vi "Make K-Points File.vi"() -> ()   [LabVIEW 2010]
uses:
  <vilib>/Analysis/NI_AALPro.lvlib
  <vilib>/Analysis/_algsub.llb/Real Vector Norm.vi
panel:
  out "K-Points File":string
  in  "Tab Control":enum32{"Automatic", "Manual"}(tab)
  in  "|G| Factor":dbl
  in  "Auto Type":T1(radio)
  in  "Shift":dbl[](array[numeric])
  in  "Lattice vector a":dbl[](array[numeric])
  in  "Lattice vector b":dbl[](array[numeric])
  in  "Lattice vector c":dbl[](array[numeric])
  in  "Symmetry":enum32{"High-Symmetry", "L-G-X", "Manual Mesh"}(radio)
  in  "# Points between":i32
  in  "Manual Type":enum32{"Reciprocal", "Cartesian"}(radio)
  in  "K-point Mesh":T2(array[cluster])
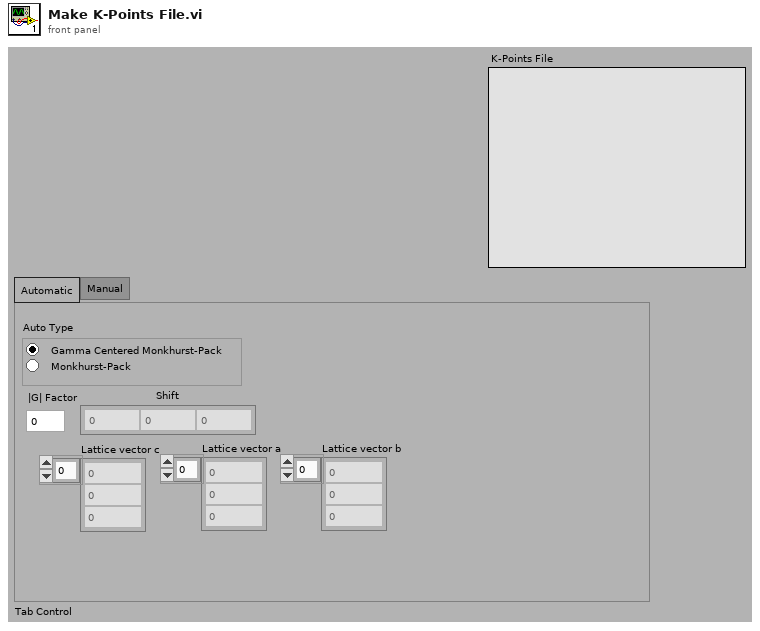
[diagram p1: front panel]
types:
  T1 = enum32{"Gamma Centered Monkhurst-Pack", "Monkhurst-Pack"}
  T2 = cluster{"Start":dbl, "End":dbl, "Step or #pts":dbl, "Style":enum16{"Linear Step", "Linear Pts", "Log Pts"}, "Parameter":string}[]
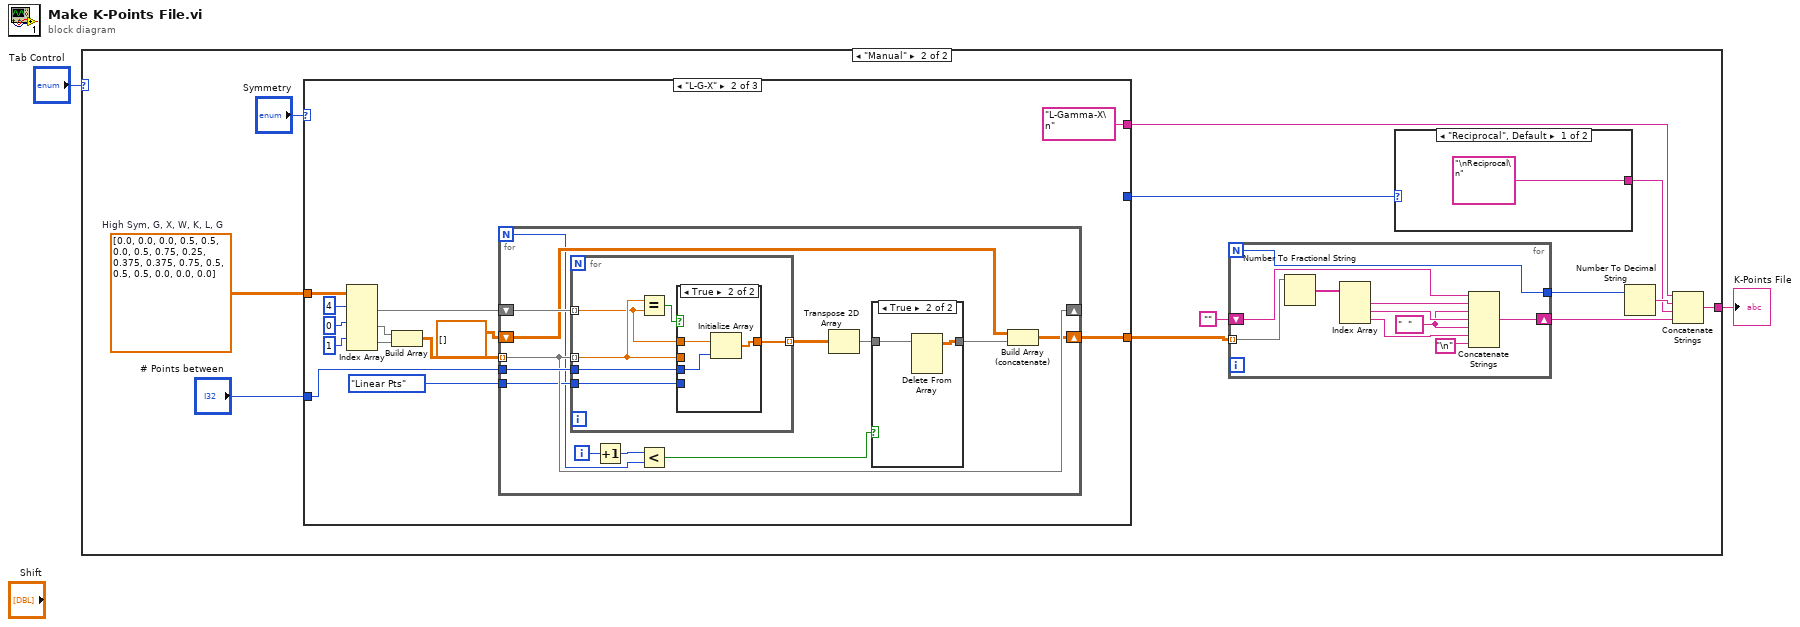
[diagram p0: block diagram]
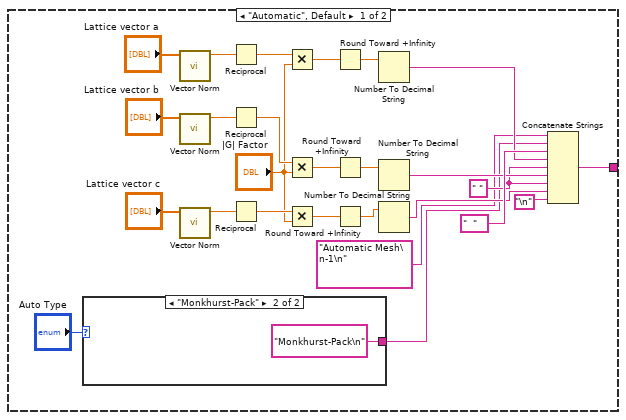
[diagram p2: hidden frame]
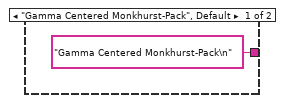
[diagram p3: hidden frame]
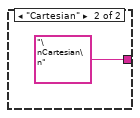
[diagram p4: hidden frame]
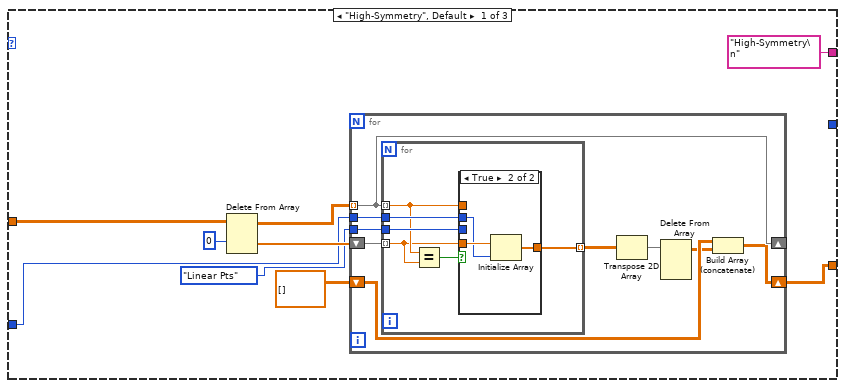
[diagram p5: hidden frame]
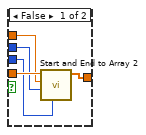
[diagram p6: hidden frame]
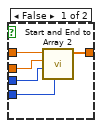
[diagram p8: hidden frame]
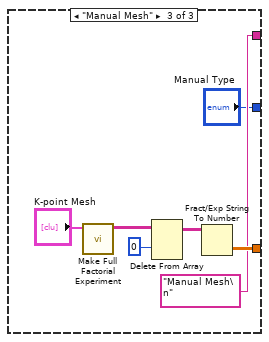
[diagram p9: hidden frame]
diagram:
  n1 = case shown="\"Manual\"" "Tab Control" {
    tunnel: [w7 w31] -> w1
    frame "Automatic", Default {
      w12 = " " ("string")
      n2 = case shown="\"Monkhurst-Pack\"" "Auto Type" {
        tunnel: ["Gamma Centered Monkhurst-Pack\n" "Monkhurst-Pack\n"] -> w8
        frame "Gamma Centered Monkhurst-Pack", Default {
        }
        frame "Monkhurst-Pack" {
        }
      }
      n3 = call-poly <vilib>:"Vector Norm.vi"("Input Vector"="Lattice vector a") -> ("norm"=w26:dbl)  [unwired: 9 in, 1 out]
      n4 = call-poly <vilib>:"Vector Norm.vi"("Input Vector"="Lattice vector b") -> ("norm"=w23:dbl)  [unwired: 9 in, 1 out]
      n5 = call-poly <vilib>:"Vector Norm.vi"("Input Vector"="Lattice vector c") -> ("norm"=w20:dbl)  [unwired: 9 in, 1 out]
      n6 = Reciprocal(x=w26) -> (1/x=w27:dbl)
      n7 = Reciprocal(x=w23) -> (1/x=w22:dbl)
      n8 = Reciprocal(x=w20) -> (1/x=w21:dbl)
      n9 = Multiply(x=w27, y="|G| Factor") -> (x*y=w25:dbl)
      n10 = Multiply(x=w22, y="|G| Factor") -> (x*y=w24:dbl)
      n11 = Multiply(x=w21, y="|G| Factor") -> (x*y=w19:dbl)
      n12 = Round Toward +Infinity(x=w25) -> (ceil(x): smallest int >= x=w18:dbl)
      n13 = Round Toward +Infinity(x=w24) -> (ceil(x): smallest int >= x=w17:dbl)
      n14 = Round Toward +Infinity(x=w19) -> (ceil(x): smallest int >= x=w16:dbl)
      n15 = Number To Decimal String(number=w18) -> (decimal integer string=w14:string)  [unwired: 1 in]
      n16 = Number To Decimal String(number=w17) -> (decimal integer string=w13:string)  [unwired: 1 in]
      n17 = Number To Decimal String(number=w16) -> (decimal integer string=w11:string)  [unwired: 1 in]
      n18 = Concatenate Strings("Automatic Mesh\n-1\n", w8, "  " ("string"), w14, w12, w13, w12, w11, "\n") -> (w7:string)
    }
    frame "Manual" {
      w41 = dbl[][] [[0.0, 0.0, 0.0], [0.5, 0.5, 0.0], [0.5, 0.75, 0.25], [0.375, 0.375, 0.75], [0.5, 0.5, 0.5], [0.0, 0.0, 0.0]]  # High Sym, G, X, W, K, L, G
      n19 = case shown="\"L-G-X\"" "Symmetry" {
        tunnel: w41 -> [w62 w89 _]
        tunnel: [w56 w96 w132] -> w39
        tunnel: "# Points between" -> [w58 w98 _]
        tunnel: ["High-Symmetry\n" "L-Gamma-X\n" "Manual Mesh\n"] -> w37
        tunnel: [_ _ "Manual Type"] -> w34
        frame "High-Symmetry", Default {
          n20 = Delete From Array(array=w62, index (row)=0) -> (deleted portion=w60:dbl[], array with subset deleted=w59:dbl[][])  [unwired: 2 in]
          n21 = for {
            shift-right: [w70] -> _
            shift-left: w60 -> [w72]
            shift-right: [w68] -> w56
            shift-left: dbl[][] [] -> [w67]
            tunnel: w59 -> [w70] mode=indexing
            tunnel: w58 -> [w71]
            tunnel: enum16{"Linear Step", "Linear Pts", "Log Pts"}."Linear Pts" ("Sweep Style") -> [w66]
            n22 = for {
              tunnel: w72 -> [w74] mode=indexing
              tunnel: w70 -> [w75] mode=indexing
              tunnel: w71 -> [w78]
              tunnel: [w77] -> w69 mode=indexing
              tunnel: w66 -> [w76]
              n23 = Equal?(x=w75, y=w74) -> (x = y?=w73:bool)
              n24 = case shown="True" w73 {
                tunnel: w74 -> [w83 w86]
                tunnel: w75 -> [w82 _]
                tunnel: w78 -> [w81 w85]
                tunnel: [w80 w84] -> w77
                tunnel: w76 -> [w79 _]
                frame False {
                  n25 = call "Start and End to Array 2.vi"("Sweep Style"=w79, "Step or # Pts"=w81, "End"=w82, "Start"=w83) -> ("Array"=w80:dbl[])  [unwired: 7 in]
                }
                frame True {
                  n26 = Initialize Array(w86, w85) -> (w84:dbl[])
                }
              }
            }
            n27 = Transpose 2D Array(2D array=w69) -> (transposed array=w65:dbl[][])
            n28 = Delete From Array(array=w65) -> (array with subset deleted=w64:dbl[][])  [unwired: 3 in, 1 out]
            n29 = Build Array (concatenate)(w67, w64) -> (w68:dbl[][])
          }
        }
        frame "L-G-X" {
          n30 = Index Array(array=w89, index (row) #1=4 ("index (row)"), index (row) #2=0 ("index (row)"), index (row) #3=1 ("index (row)")) -> (element #1=w88:dbl[], element #2=w91:dbl[], element #3=w90:dbl[])  [unwired: 3 in]
          n31 = Build Array(w91, w90) -> (w87:dbl[][])
          n32 = for {
            N -> [w101]
            shift-right: [w110] -> _
            shift-left: w88 -> [w112]
            shift-right: [w108] -> w96
            shift-left: dbl[][] [] -> [w107]
            tunnel: w87 -> [w110] mode=indexing
            tunnel: w98 -> [w111]
            tunnel: enum16{"Linear Step", "Linear Pts", "Log Pts"}."Linear Pts" ("Sweep Style") -> [w106]
            i -> [w103]
            n33 = for {
              tunnel: w112 -> [w117] mode=indexing
              tunnel: w110 -> [w118] mode=indexing
              tunnel: w111 -> [w121]
              tunnel: [w120] -> w109 mode=indexing
              tunnel: w106 -> [w119]
              n34 = Equal?(x=w118, y=w117) -> (x = y?=w116:bool)
              n35 = case shown="True" w116 {
                tunnel: w117 -> [w126 w129]
                tunnel: w118 -> [w125 _]
                tunnel: w121 -> [w124 w128]
                tunnel: [w123 w127] -> w120
                tunnel: w119 -> [w122 _]
                frame False {
                  n36 = call "Start and End to Array 2.vi"("Sweep Style"=w122, "Step or # Pts"=w124, "End"=w125, "Start"=w126) -> ("Array"=w123:dbl[])  [unwired: 7 in]
                }
                frame True {
                  n37 = Initialize Array(w129, w128) -> (w127:dbl[])
                }
              }
            }
            n38 = Increment(x=w103) -> (x+1=w102:i32)
            n39 = Less?(x=w102, y=w101) -> (x < y?=w100:bool)
            n40 = Transpose 2D Array(2D array=w109) -> (transposed array=w105:dbl[][])
            n41 = case shown="True" w100 {
              tunnel: w105 -> [w113 w115]
              tunnel: [w113 w114] -> w104
              frame False {
              }
              frame True {
                n42 = Delete From Array(array=w115) -> (array with subset deleted=w114:dbl[][])  [unwired: 3 in, 1 out]
              }
            }
            n43 = Build Array (concatenate)(w107, w104) -> (w108:dbl[][])
          }
        }
        frame "Manual Mesh" {
          n44 = call "Make Full Factorial Experiment.vi"("Array of Array Settings"="K-point Mesh") -> ("Full Factorial Design"=w135:string[][])  [unwired: 10 in]
          n45 = Delete From Array(array=w135, index (row)=0) -> (array with subset deleted=w133:string[][])  [unwired: 2 in, 1 out]
          n46 = Fract/Exp String To Number(string=w133) -> (number=w132:dbl[][])  [unwired: 3 in, 1 out]
        }
      }
      n47 = for {
        N -> [w45]
        tunnel: w39 -> [w54] mode=indexing
        shift-right: [w47] -> w32
        shift-left: "" -> [w46]
        tunnel: [w45] -> w36
        w50 = "  "
        n48 = Number To Fractional String(number=w54) -> (F-format string=w53:string[])  [unwired: 3 in]
        n49 = Index Array(array=w53) -> (element #1=w52:string, element #2=w51:string, element #3=w49:string)  [unwired: 3 in]
        n50 = Concatenate Strings(w46, w52, w50, w51, w50, w49, "\n") -> (w47:string)
      }
      n51 = case shown="\"Reciprocal\", Default" w34 {
        tunnel: ["\nReciprocal\n" "\nCartesian\n"] -> w33
        frame "Reciprocal", Default {
        }
        frame "Cartesian" {
        }
      }
      n52 = Number To Decimal String(number=w36) -> (decimal integer string=w35:string)  [unwired: 1 in]
      n53 = Concatenate Strings(w37, w35, w33, w32) -> (w31:string)
    }
  }
  "K-Points File" <- w1
